vi "TimeInterpRotation_Clear.vi"(11 "in TimeInterpRotation":T1 {"RotationValues"."SIN" format="%13.4f"; "RotationValues"."COS" format="%13.4f"; "RotationValues"."VALUE" format="%13.4f"}) -> (3 "out TimeInterpRotation":T1 {"RotationValues"."SIN" format="%13.4f"; "RotationValues"."COS" format="%13.4f"; "RotationValues"."VALUE" format="%13.4f"})   [LabVIEW 2019, in "Trajectory_Library.lvlib"]
doc: "Inputs:\n - \n\nOutputs:\n - Function Generator -- Created data structure"
uses:
  Trajectory_Library.lvlib
  ROTATION2D.ctl
  TIME_INTERPOLATABLE_ROTATION.ctl
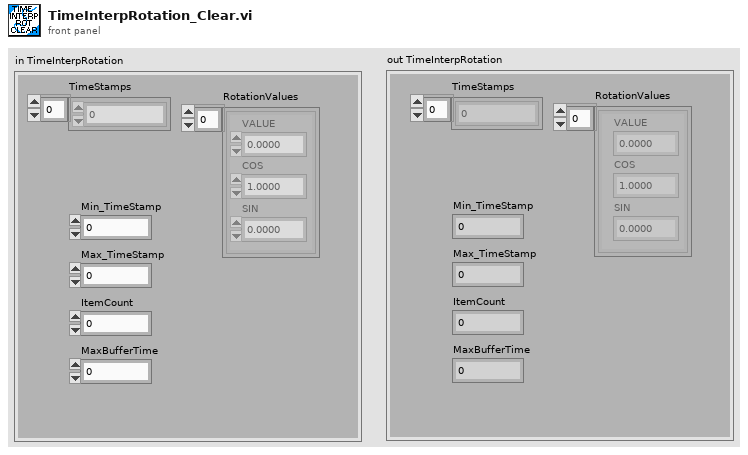
[diagram p1: front panel]
types:
  T1 = typedef "Trajectory_Library.lvlib/TIME_INTERPOLATABLE_ROTATION.ctl" = cluster{"TimeStamps":dbl[], "RotationValues":T2[], "Min_TimeStamp":dbl, "Max_TimeStamp":dbl, "ItemCount":i32, "MaxBufferTime":dbl}
  T2 = typedef "Trajectory_Library.lvlib/ROTATION2D.ctl" = cluster{"VALUE":dbl, "COS":dbl, "SIN":dbl}
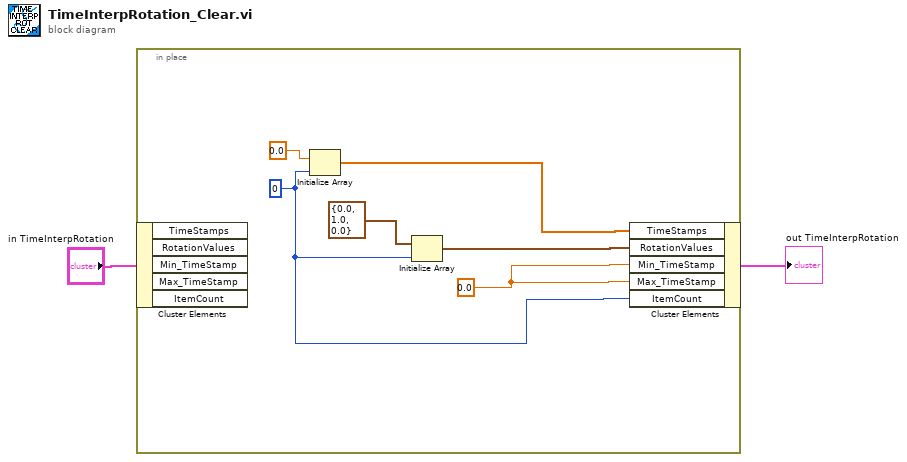
[diagram p0: block diagram]
diagram:
  n1 = in-place {
    w4 = 0.0 ("X")
    w3 = 0 ("dimension size")
    n2 = in-place-cluster #1("in TimeInterpRotation") -> ()  [unwired: 5 out]
    n3 = Initialize Array(0.0 ("element"), w3) -> (w6:dbl[])
    n4 = Initialize Array(T2 {"VALUE"=0.0, "COS"=1.0, "SIN"=0.0} ("ROTATION"), w3) -> (w5:T2[])
    n5 = in-place-cluster #1("TimeStamps"=w6, "RotationValues"=w5, "Min_TimeStamp"=w4, "Max_TimeStamp"=w4, "ItemCount"=w3) -> (→"out TimeInterpRotation":T1)
  }
